vi "Launch Topic.vi"(7 "Include Initial Value? (F)":bool, 9 "Type":variant, 10 "Datum Name":string, 11 "Mediator in":refnum<class "Mediator.lvclass">) -> (0 "error out":errorcluster, 2 "New Topic Enqueuer":refnum<class "Message Enqueuer.lvclass">, 3 "Mediator out":refnum<class "Mediator.lvclass">)   [LabVIEW 2017, in "Mediator.lvlib" / "Mediator.lvclass"]
uses:
  Mediator.lvclass
  C:/Program Files (x86)/National Instruments/LabVIEW 2017/vi.lib/ActorFramework/Actor/Actor.lvclass
  <vilib>/ActorFramework/Message Enqueuer/Message Enqueuer.lvclass
  SubscriptionPolicy/BasicSubscription/BasicSubscription.lvclass/BasicSubscription.ctl
  Mediator.lvclass/Mediator.ctl
  Transport/ActorMessageTransport/ActorMessageTransport.lvclass/ActorMessageTransport.ctl
  Topic/Topic.lvclass/Topic.ctl
  TopicLookupTable/TopicLookupTable.lvclass/TopicLookupTable.ctl
  Topic Messages/Add Topic Subscriber Msg/Add Topic Subscriber Msg.lvclass/Add Topic Subscriber Msg.ctl
  <vilib>/ActorFramework/Message Enqueuer/Message Enqueuer.lvclass/Message Enqueuer.ctl
  Topic/Read Topic Info.vi
  <vilib>/ActorFramework/Message Enqueuer/Enqueue.vi
  <vilib>/ActorFramework/Actor/Read Self Enqueuer.vi
  <vilib>/ActorFramework/Message Enqueuer/Init from Existing Queue.vi
  SubscriptionPolicy/BasicSubscription/BasicSubscription.lvclass
  C:/Git/mva-framework/Source/Framework/IMediator/ISubscriptionPolicy/ISubscriptionPolicy.lvclass
  Topic/Topic.lvclass
  Transport/ActorMessageTransport/ActorMessageTransport.lvclass
  C:/Git/mva-framework/Source/Framework/IMediator/ITransport/ITransport.lvclass
  Topic Messages/Add Topic Subscriber Msg/Add Topic Subscriber Msg.lvclass
  C:/Program Files (x86)/National Instruments/LabVIEW 2017/vi.lib/ActorFramework/Message/Message.lvclass
  Transport/ActorMessageTransport/Notification Msg/Write Notification Msg Return Info.vi
  <vilib>/ActorFramework/Message Priority Queue/Priority Enqueue.vi
  <vilib>/ActorFramework/Actor/Actor.lvclass
  TopicLookupTable/TopicLookupTable.lvclass
  IMediator/ISubscriptionPolicy/ISubscriptionPolicy.lvclass
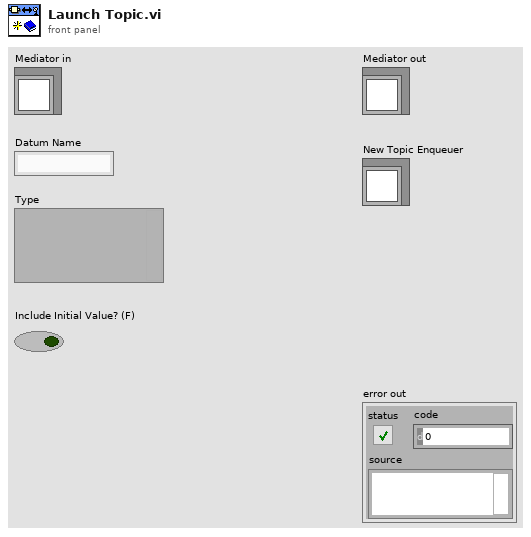
[diagram p1: front panel]
types:
  T1 = typedef "IMediator.lvlib/ISubscriptionPolicy.lvclass/ISubscriptionPolicy Reference.ctl" = refnum<data-value>
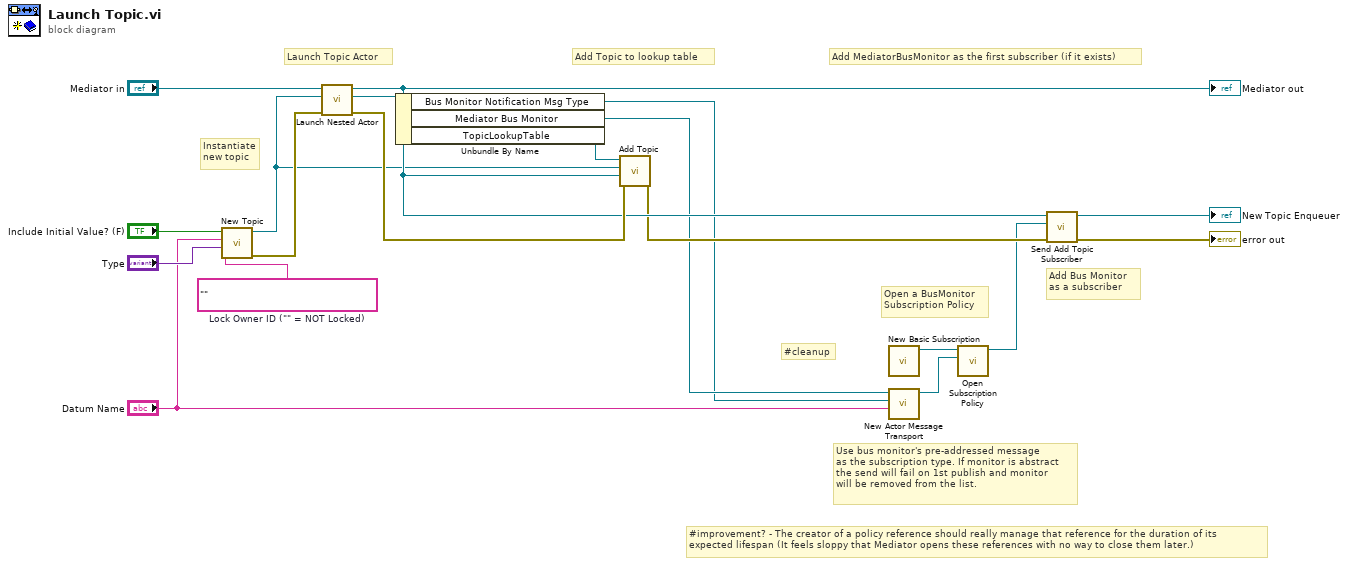
[diagram p0: block diagram]
diagram:
  w5 = ""  # Lock Owner ID ("" = NOT Locked)
  # "#cleanup"
  # "Open a BusMonitor\nSubscription Policy"
  # "Add Bus Monitor\nas a subscriber"
  # "Use bus monitor's pre-addressed message\nas the subscription type. If monitor is abstract\nthe send will fail on 1st publish and monitor\nwill be removed from the list."
  # "#improvement? - The creator of a policy reference should really manage that reference for the duration of its\nexpected lifespan (It feels sloppy that Mediator opens these references with no way to close them later.)"
  # "Add MediatorBusMonitor as the first subscriber (if it exists)"
  # "Launch Topic Actor"
  # "Add Topic to lookup table"
  # "Instantiate\nnew topic"
  n1 = call "New Topic.vi"("Lock Owner ID (\"\" = NOT Locked)"=w5, "New Topic Data"="Type", "Name"="Datum Name", "Use Type Input As Initial Value?"="Include Initial Value? (F)") -> ("error out"=w14:errorcluster, "Topic out"=w13:refnum<class "Topic.lvclass">)  [unwired: 6 in]
  n2 = call <vilib>:"Launch Nested Actor.vi"("error in (no error)"=w14, "Nested Actor"=w13, "Caller Actor in"="Mediator in") -> ("error out"=w17:errorcluster, "Nested Actor's Enqueuer"=w15:refnum<class "Message Enqueuer.lvclass">, "Caller Actor out"=w9:refnum<class "Mediator.lvclass">)  [unwired: 6 in]
  "Mediator out" <- w9
  n3 = Unbundle By Name(w9) -> ("Bus Monitor Notification Msg Type"=w1:refnum<class "Notification Msg.lvclass">, "Mediator Bus Monitor"=w7:refnum<class "Message Enqueuer.lvclass">, "TopicLookupTable"=w12:refnum<data-value>)
  n4 = call "Add Topic.vi"("error in (no error)"=w17, "Topic Enqueuer"=w15, "Topic Object"=w13, "TopicLookupTable"=w12) -> ("error out"=w11:errorcluster)  [unwired: 5 in, 2 out]
  n5 = call "New Basic Subscription.vi"() -> ("BasicSubscription Out"=w3:refnum<class "BasicSubscription.lvclass">)  [unwired: 11 in]
  n6 = call "New Actor Message Transport.vi"("Datum Name"="Datum Name", "Desired Notification Msg (Type)"=w1, "Message Enqueuer in"=w7) -> ("ActorMessageTransport"=w4:refnum<class "ActorMessageTransport.lvclass">)  [unwired: 7 in, 1 out]
  n7 = call "Open Subscription Policy.vi"("Transport"=w4, "SubscriptionPolicy"=w3) -> ("Subscription Policy"=w2:T1)  [unwired: 8 in, 1 out]
  n8 = call "Send Add Topic Subscriber.vi"("error in (no error)"=w11, "Subscription Policy"=w2, "Message Enqueuer"=w15) -> ("error out"=→"error out":errorcluster, "Message Enqueuer out"=→"New Topic Enqueuer":refnum<class "Message Enqueuer.lvclass">)  [unwired: 7 in]
